vi "pull.vi"(8 "error in (no error)":errorcluster caption="错误输入（无错误）", 9 "local file path":path caption="本地文件路径", 10 "更新包远端地址":string="/UP/OneStation/V4/一体化微型水质监测站.exe", 11 "WebDAV client 输入":refnum<class "WebDAV client.lvclass">) -> (0 "error out":errorcluster caption="错误输出", 3 "WebDAV client 输出":refnum<class "WebDAV client.lvclass">)   [LabVIEW 2016, in "数据传输系统-03.lvlib" / "update.lvlib" / "WebDAV client.lvclass"]
uses:
  WebDAV client.lvclass
  System.Web
  WebDAV client.lvclass/WebDAV client.ctl
  <vilib>/WebDAVClient/Advanced/Multi Event/Asynchronous Get File.vi
  <vilib>/WebDAVClient/NI_WebDAV.lvlib
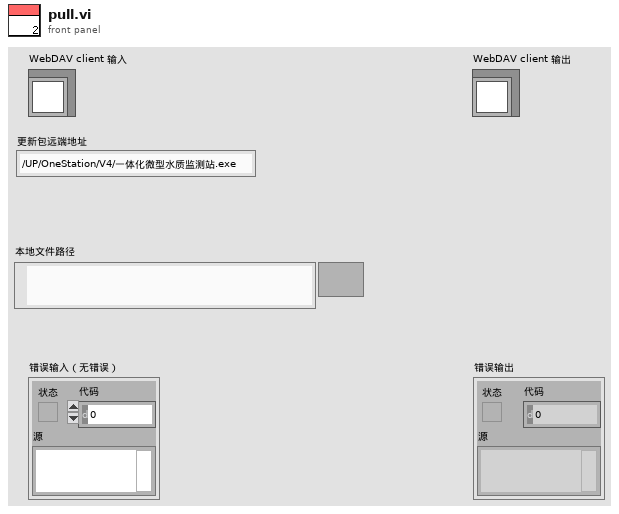
[diagram p1: front panel]
types:
  T1 = typedef "NI_WebDAV.lvlib/Asynchronous Session Handle.ctl" = refnum<k1>
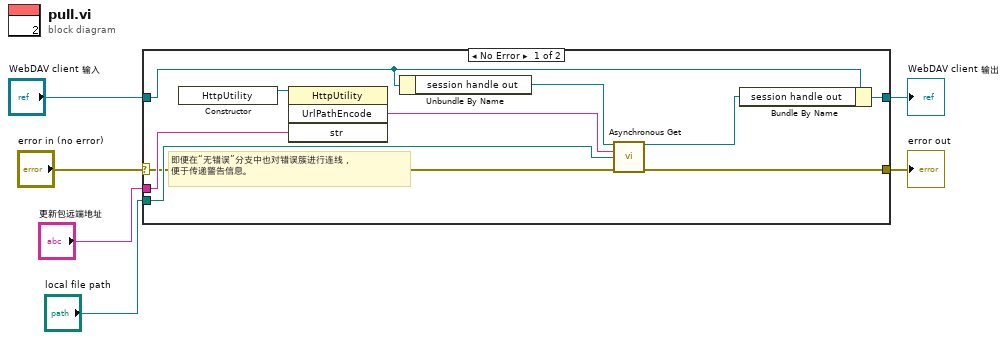
[diagram p0: block diagram]
diagram:
  n1 = case shown="No Error" "error in (no error)" {
    selector: "error in (no error)" -> [w8 w18]
    tunnel: [w7 w18] -> w5
    tunnel: [w9 w17] -> w3
    tunnel: "WebDAV client 输入" -> [w11 w17]
    tunnel: "更新包远端地址" -> [w14 _]
    tunnel: "local file path" -> [w12 _]
    frame No Error {
      # "即便在“无错误”分支中也对错误簇进行连线，\n便于传递警告信息。"
      n2 = constructor class="HttpUtility"() -> (reference out=w15:refnum<k24>)  [unwired: 3 in, 2 out]
      n3 = invoke class="HttpUtility" method="UrlPathEncode"(reference=w15, "str"=w14) -> ("UrlPathEncode"=w13:string)  [unwired: 2 in, 3 out]
      n4 = Unbundle By Name(w11) -> ("session handle out"=w16:T1)
      n5 = call-poly <vilib>:"Asynchronous Get.vi"("session handle"=w16, "relative uri"=w13, "local file path"=w12, "error in (no error)"=w8) -> ("session handle out"=w10:T1, "error out"=w7:errorcluster)  [unwired: 8 in, 2 out]
      n6 = Bundle By Name(cluster=w11, "session handle out"=w10) -> (w9:refnum<class "WebDAV client.lvclass">)
    }
    frame Error {
    }
  }
  "error out" <- w5
  "WebDAV client 输出" <- w3
